vi "Check Connection.vi"(4 "local port (0)":u16, 6 "timeout [ms]":i32=100, 8 "error in (no error)":errorcluster, 9 "remote port":u16, 10 "ip address":string, 11 "GenNet Protocol in":refnum<class "GenNet Protocol.lvclass">) -> (0 "error out":errorcluster, 3 "GenNet Protocol out":refnum<class "GenNet Protocol.lvclass">)   [LabVIEW 2022 SP3, in "hse-gennet.lvlib" / "GenNet Protocol.lvclass"]
doc: "____\nHAMPEL SOFTWARE ENGINEERING v3.8.0 (2023-12-18 14:41)"
uses:
  GenNet Protocol.lvclass
  GenNet Protocol.lvclass/GenNet Protocol.ctl
  Set Connection ID.vi
  Get Connection ID.vi
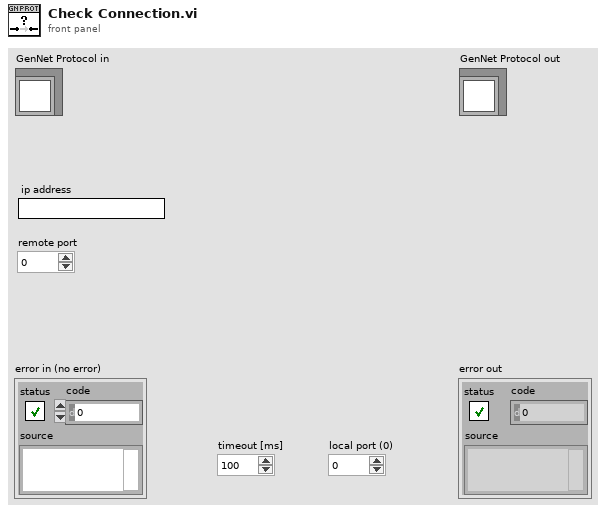
[diagram p1: front panel]
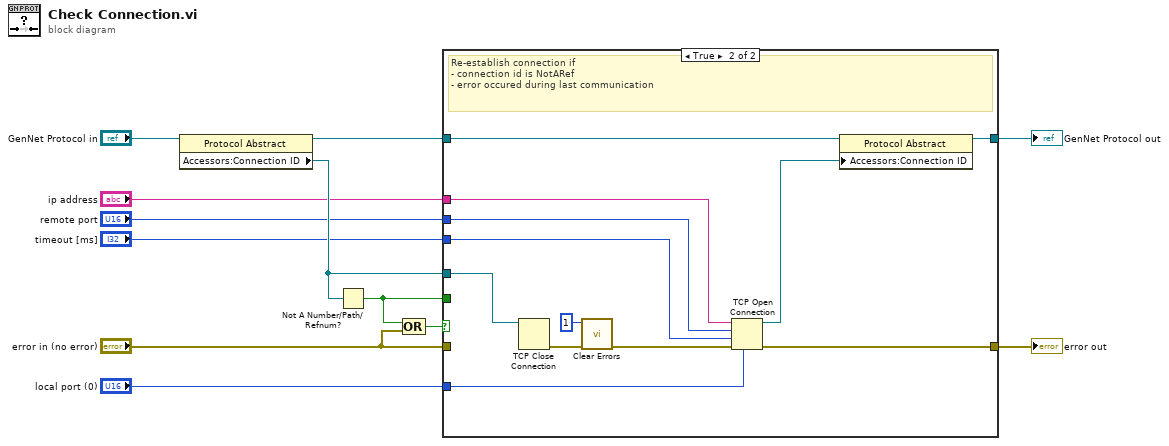
[diagram p0: block diagram]
diagram:
  n1 = property class="Protocol Abstract"(reference="GenNet Protocol in") -> (reference out=w9:refnum<class "GenNet Protocol.lvclass">, "Accessors:Connection ID"=w10:refnum<k5>)  [unwired: 1 in, 1 out]
  n2 = Not A Number/Path/Refnum?(number/path/refnum=w10) -> (NaN/Path/Refnum?=w11:bool)
  n3 = Compound Arithmetic op=OR(w11, "error in (no error)") -> (w12:bool)
  n4 = case shown="True" w12 {
    tunnel: [w14 w25] -> w1
    tunnel: "error in (no error)" -> [w14 _]
    tunnel: "local port (0)" -> [_ w24]
    tunnel: "timeout [ms]" -> [_ w23]
    tunnel: "remote port" -> [_ w22]
    tunnel: "ip address" -> [_ w21]
    tunnel: w10 -> [_ w18]
    tunnel: w11 -> [_ _]
    tunnel: w9 -> [w13 w17]
    tunnel: [w13 w16] -> w7
    frame False {
      # "Use existing connection"
    }
    frame True {
      # "Re-establish connection if \n- connection id is NotARef\n- error occured during last communication"
      n5 = TCP Close Connection(connection ID=w18) -> (error out=w26:errorcluster)  [unwired: 1 in, 2 out]
      n6 = call <vilib>:"Clear Errors.vi"("error in (no error)"=w26, "specific error code to clear (0: all)"=1) -> ("error out"=w20:errorcluster)  [unwired: 4 in, 1 out]
      n7 = TCP Open Connection(address=w21, remote port or service name=w22, timeout ms (60000)=w23, local port=w24, error in (no error)=w20) -> (connection ID=w15:refnum<k5>, error out=w25:errorcluster)
      n8 = property class="Protocol Abstract"(reference=w17, "Accessors:Connection ID"=w15) -> (reference out=w16:refnum<class "GenNet Protocol.lvclass">)  [unwired: 1 in, 1 out]
    }
  }
  "error out" <- w1
  "GenNet Protocol out" <- w7
